vi "WPI_PotentiometerOpen.vi"(8 "error in (no error)":errorcluster, 9 "Invert Output":bool, 10 "Analog Channel":T1) -> (0 "error out":errorcluster, 3 "PotDevRef":T2={"DevStatus"={"status"=FALSE, "code"=0, "source"=""}, "Analog Channel"=enum."Invalid", "Invert Output"=FALSE})   [LabVIEW 2017]
doc: "Opens a reference to the potentiometer you specify. You must open a reference before using any other Potentiometer VIs.\n\nThis software is licensed. Open the labview\\readme\\WPI Robotics Library Open Source License.txt file for more information."
uses:
  <vilib>/Rock Robotics/WPI/Potentiometer/WPI_PotentiometerDevRef.ctl
  <vilib>/Rock Robotics/SystemInterfaces/AI/FPGA_AIChannel.ctl
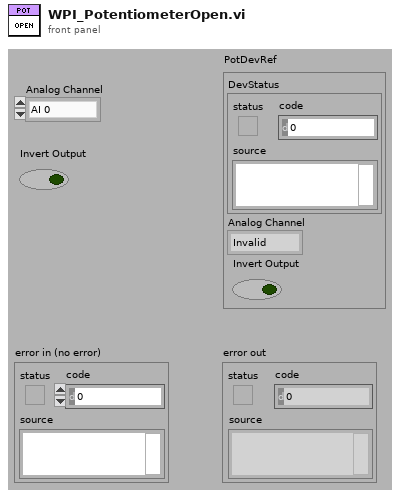
[diagram p1: front panel]
types:
  T1 = typedef "FPGA_AIChannel.ctl" = enum8{"AI 0", "AI 1", "AI 2", "AI 3", "AI MXP 0", "AI MXP 1", "AI MXP 2", "AI MXP 3", "Invalid"}
  T2 = typedef "WPI_PotentiometerDevRef.ctl" = cluster{"DevStatus":errorcluster, "Analog Channel":T1, "Invert Output":bool}
  T3 = typedef "WPI_AnalogChannelDevRef.ctl" = cluster{"DevStatus":errorcluster, "Analog Channel":T1}
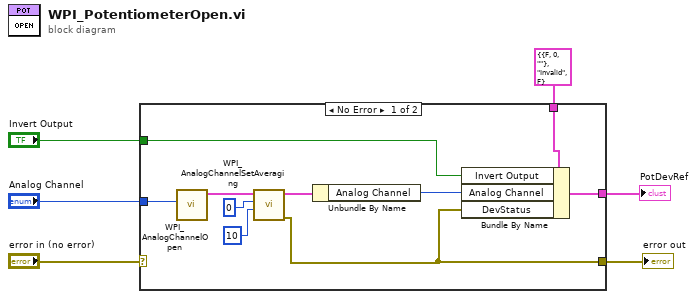
[diagram p0: block diagram]
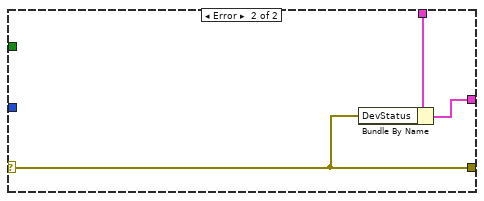
[diagram p2: hidden frame]
diagram:
  n1 = case shown="No Error" "error in (no error)" {
    selector: "error in (no error)" -> [_ w17]
    tunnel: T2 {"DevStatus"={"status"=FALSE, "code"=0, "source"=""}, "Analog Channel"=enum."Invalid", "Invert Output"=FALSE} ("PotDevRef") -> [w16 w19]
    tunnel: [w15 w18] -> w6
    tunnel: "Analog Channel" -> [w13 _]
    tunnel: [w11 w17] -> w3
    tunnel: "Invert Output" -> [w7 _]
    frame No Error {
      n2 = call <vilib>:"WPI_AnalogChannelOpen.vi"("Analog Channel"=w13) -> ("AIDeviceRef"=w14:T3)  [unwired: 9 in, 1 out]
      n3 = call <vilib>:"WPI_AnalogChannelSetAveraging.vi"("OversampleBits"=u8 10, "AverageBits"=u8 0, "AIDeviceRef"=w14) -> ("error out"=w11:errorcluster, "AIDeviceRef"=w10:T3)  [unwired: 7 in]
      n4 = Unbundle By Name(w10) -> ("Analog Channel"=w9:T1)
      n5 = Bundle By Name(cluster=w16, "Invert Output"=w7, "Analog Channel"=w9, "DevStatus"=w11) -> (w15:T2)
    }
    frame Error {
      n6 = Bundle By Name(cluster=w19, "DevStatus"=w17) -> (w18:T2)
    }
  }
  "PotDevRef" <- w6
  "error out" <- w3
